vi "5060_set_all_outputs.vi"(1 "Address (Main, Sub reqd.)":T1, 2 "Digital output state byte":u16 max=63 format="%.0b") -> (3 "Reply":string, 6 "Good Reply":bool)   [LabVIEW 2010]
uses:
  ADAM Client/Sub VIs/ADAM Controls/Address.ctl
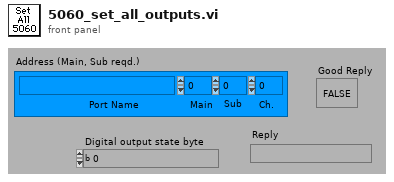
[diagram p1: front panel]
types:
  T1 = typedef "Address.ctl" = cluster{"Main":i32, "Ch.":i32, "Sub":i32, "Port Name":string}
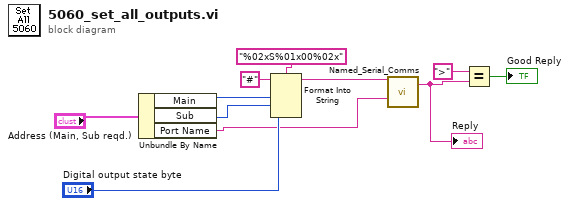
[diagram p0: block diagram]
diagram:
  n1 = Unbundle By Name("Address (Main, Sub reqd.)") -> ("Main"=w10:i32, "Sub"=w11:i32, "Port Name"=w2:string)
  n2 = Format Into String(format string="%02xS%01x00%02x", initial string="#", w10, w11, "Digital output state byte") -> (resulting string=w7:string)  [unwired: 1 in, 1 out]
  n3 = call "Named_Serial_Comms.vi"("Write String"=w7, "Port Name"=w2) -> ("Read"=w1:string)  [unwired: 10 in, 3 out]
  "Reply" <- w1
  n4 = Equal?(x=">", y=w1) -> (x = y?=→"Good Reply":bool)
